vi "USBClient1Pub.vi"() -> ()   [LabVIEW 2018]
uses:
  <vilib>/daq.io/MQTT LabVIEW Client/Controls/Connect_Flags.ctl
  <vilib>/daq.io/MQTT LabVIEW Client/Controls/QoS.ctl
  <vilib>/daq.io/MQTT LabVIEW Client/Controls/DUP_Flag.ctl
  <vilib>/daq.io/MQTT LabVIEW Client/Controls/Retain_Flag.ctl
  <vilib>/DAQmx/read.llb/DAQmx Read (Analog DBL 1Chan 1Samp).vi
  <vilib>/DAQmx/create/channels.llb/DAQmx Create Channel (AI-Voltage-Basic).vi
  <vilib>/DAQmx/miscellaneous.llb/DAQmx Fill In Error Info.vi
  <vilib>/daq.io/MQTT LabVIEW Client/MQTT_Functions.lvlib
panel:
  in  "stop":bool
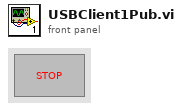
[diagram p1: front panel]
types:
  T1 = typedef "MQTT_Functions.lvlib/QoS.ctl" = enum8{"At most once", "At least once", "Exactly once", "Reserved"}
  T2 = typedef "MQTT_Functions.lvlib/Retain_Flag.ctl" = bool
  T3 = typedef "MQTT_Functions.lvlib/DUP_Flag.ctl" = bool
  T4 = cluster{"QoS":T1, "DUP":T3, "Retain":T2, "Keep Alive (sec)":u16}
  T5 = typedef "MQTT_Functions.lvlib/Connect_Flags.ctl" = cluster{"user name":bool, "password":bool, "will retain":bool, "will flag":bool, "clean session":bool, "reserved":bool, "will QoS":T1}
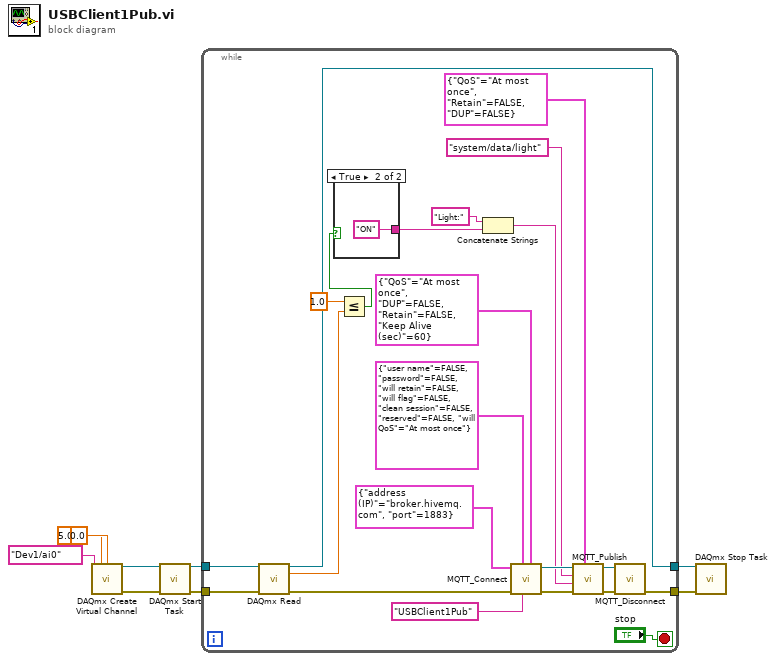
[diagram p0: block diagram]
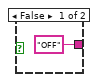
[diagram p2: hidden frame]
diagram:
  n1 = call-poly <vilib>:"DAQmx Create Virtual Channel.vi"("maximum value"=5.0, "minimum value"=0.0, "physical channels"=tag "Dev1/ai0") -> ("task out"=w9:refnum<k21>, "error out"=w8:errorcluster)  [unwired: 11 in]
  n2 = call <vilib>:"DAQmx Start Task.vi"("task/channels in"=w9, "error in"=w8) -> ("task out"=w7:refnum<k21>, "error out"=w6:errorcluster)  [unwired: 12 in]
  n3 = while {
    tunnel: w7 -> [w31]
    tunnel: w6 -> [w30]
    tunnel: [w29] -> w4
    tunnel: [w13] -> w5
    stop <- "stop" stop-if-true
    n4 = call-poly <vilib>:"DAQmx Read.vi"("task/channels in"=w31, "error in"=w30) -> ("task out"=w29:refnum<k21>, "data"=w12:dbl, "error out"=w27:errorcluster)  [unwired: 11 in]
    n5 = Less Or Equal?(x=1.0, y=w12) -> (x <= y?=w10:bool)
    n6 = case shown="True" w10 {
      tunnel: ["OFF" "ON"] -> w18
      frame False {
      }
      frame True {
      }
    }
    n7 = Concatenate Strings("Light:" ("Message to be published"), w18) -> (w17:string)
    n8 = call <vilib>:"MQTT_Connect.vi"("Connect Meta"=T4 {"QoS"=enum."At most once", "DUP"=FALSE, "Retain"=FALSE, "Keep Alive (sec)"=60}, "Client ID"="USBClient1Pub", "Connect Flags"=T5 {"user name"=FALSE, "password"=FALSE, "will retain"=FALSE, "will flag"=FALSE, "clean session"=FALSE, "reserved"=FALSE, "will QoS"=enum."At most once"}, "error in (no error)"=w27, "MQTT Broker"=cluster{"address (IP)":string, "port":u16} {"address (IP)"="broker.hivemq.com", "port"=1883}) -> ("error out"=w22:errorcluster, "connection ID out"=w21:refnum<k5>)  [unwired: 4 in, 1 out]
    n9 = call <vilib>:"MQTT_Publish.vi"("Publish Meta"=cluster{"QoS":T1, "Retain":T2, "DUP":T3} {"QoS"=enum."At most once", "Retain"=FALSE, "DUP"=FALSE}, "error in (no error)"=w22, "Message to be published"=w17, "Topic"="system/data/light", "connection ID"=w21) -> ("error out"=w15:errorcluster, "connection ID out"=w14:refnum<k5>)  [unwired: 5 in]
    n10 = call <vilib>:"MQTT_Disconnect.vi"("error in (no error)"=w15, "connection ID"=w14) -> ("error out"=w13:errorcluster)  [unwired: 9 in]
  }
  n11 = call <vilib>:"DAQmx Stop Task.vi"("task/channels in"=w4, "error in"=w5) -> ()  [unwired: 12 in, 2 out]
